vi "PH_Beckhoff_StepMot.ProcPeriodic.vi"(0 "i ref in":refnum<vi>, 3 "ms timeout (10000)":i32=10000, 5 "error in (no error)":errorcluster) -> (14 "i ref out":refnum<vi>, 17 "timed out":bool, 19 "error out":errorcluster)   [LabVIEW 2014, in "PH_Beckhoff_StepMot.lvlib"]
doc: "This method serves to periodically do things like reading values from the HW. Methods that should be executed periodically should be called from THIS methode. Add code here."
uses:
  PH_Beckhoff_StepMot.lvlib
  PH_Beckhoff/PH_Beckhoff.lvlib
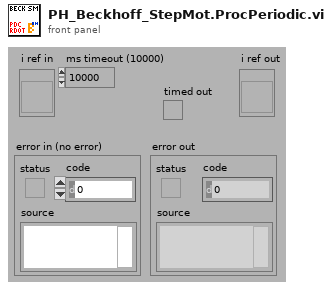
[diagram p1: front panel]
types:
  T1 = typedef "PH_Beckhoff.lvlib/PH_Beckhoff.i attribute.ctl" = cluster{"GUI Refs":T2, "operation?":bool, "Default Prdc Interval":i32, "Connection":T3, "AMS Net ID":T4, "Klemmencluster: # of":T5, "Values":T6, "IP":string, "Description":string, "configured?":bool, "Change Manager":cluster{"Detemination wanted?":bool, "Values changed at":cluster{"Sonderklemmen Inputs":i32[], "Analog Inputs":i32[], "Analog Outputs":i32[], "Digital Inputs":i32[], "Digital Outputs":i32[]}}, "Difference to handle an analog input as change":u32}
  T2 = typedef "PH_Beckhoff.lvlib/PH_Beckhoff.GUI Refs.ctl" = cluster{"ADS Error":refnum<vi>, "Values":refnum<vi>, "configured?":refnum<vi>, "Connection":refnum<vi>, "IP":refnum<vi>, "Prdc Int [ms]":refnum<vi>}
  T3 = typedef "PH_Beckhoff.lvlib/PH_Beckhoff.Connectivity.ctl" = cluster{"DLL?":bool, "Port?":bool, "Client?":bool, "Ping?":bool, "unsuccessful Pings":u32}
  T4 = typedef "Beckhoff - Driver np.lvlib/Beckhoff Access.ctl" = cluster{"DLL path":path, "AMS Net ID":cluster{"1st # of IP":u8, "2nd # of IP":u8, "3rd # of IP":u8, "4th # of IP":u8, "In Port":u8, "Out Port":u8}}
  T5 = typedef "Beckhoff - Driver np.lvlib/Klemmendeclarer.ctl" = cluster{"Offset due to Sonderklemms":u32, "analog Inputs":u32, "analog Outputs":u32, "digital Input Bits":u32, "digital Output Bits":u32}
  T6 = typedef "PH_Beckhoff.lvlib/PH_Beckhoff.Values.ctl" = cluster{"Sonderklemmen Inputs":T7, "Analog Inputs":T8, "Analog Outputs":T10, "Digital Inputs":T11, "Digital Outputs":T12}
  T7 = typedef "PH_Beckhoff.lvlib/PH_Beckhoff.Sonderklemmen Inputs.ctl" = cluster{"Total Length":u32, "Name":string, "Value":u64, "Quality":bool, "Service ID":i32, "Offset":u32, "Length":u32}[]
  T8 = typedef "PH_Beckhoff.lvlib/PH_Beckhoff.Analog Inputs.ctl" = cluster{"Name":string, "Value":u32, "Quality":bool, "Service ID":i32, "Sca Type":T9}[]
  T9 = typedef "PH_Beckhoff.lvlib/PH_Beckhoff.Scaling Type.ctl" = enum16{"none", "0 ... 15 Bit -> 0 ... 5", "0 ... 15 Bit -> 0 ... 10", "0 ... 15 Bit -> 0 ... 25", "0 ... 15 Bit -> 4 ... 20", "0 ... 15 Bit -> 0 ... 1", "0 ... 15 Bit -> 0 ... 20000", "0 ... 15 Bit -> 0 ... 24000"}
  T10 = typedef "PH_Beckhoff.lvlib/PH_Beckhoff.Analog Outputs.ctl" = cluster{"Name":string, "Value":u32, "Quality":bool, "Wanted Value":u32, "Service ID":i32, "Sca Type":T9}[]
  T11 = typedef "PH_Beckhoff.lvlib/PH_Beckhoff.Digital Inputs.ctl" = cluster{"Name":string, "Value":bool, "Quality":bool, "Service ID":i32, "inverted?":bool}[]
  T12 = typedef "PH_Beckhoff.lvlib/PH_Beckhoff.Digital Outputs.ctl" = cluster{"Name":string, "Value":bool, "Quality":bool, "Wanted Value":bool, "Service ID":i32, "inverted?":bool}[]
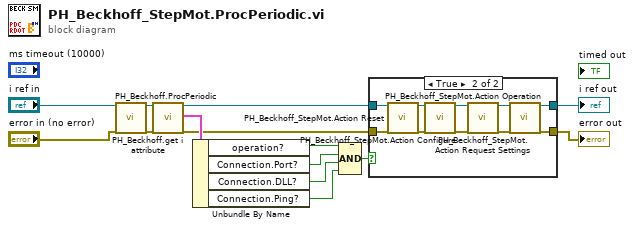
[diagram p0: block diagram]
diagram:
  n1 = call "PH_Beckhoff.ProcPeriodic.vi"("i ref in"="i ref in", "error in (no error)"="error in (no error)") -> ("i ref out"=w2:refnum<vi>, "error out"=w1:errorcluster)  [unwired: 15 in, 1 out]
  n2 = call "PH_Beckhoff.get i attribute.vi"("i ref in"=w2, "error in (no error)"=w1) -> ("i ref out"=w10:refnum<vi>, "i attribute"=w12:T1, "error out"=w9:errorcluster)  [unwired: 15 in]
  n3 = Unbundle By Name(w12) -> ("operation?"=w6:bool, "Connection.Port?"=w8:bool, "Connection.DLL?"=w7:bool, "Connection.Ping?"=w5:bool)
  n4 = Compound Arithmetic op=AND(w6, w8, w7, w5) -> (w11:bool)
  n5 = case "Constructor finished, DLL and Client found, port opened and hardware pinged?" shown="True" w11 {
    tunnel: w9 -> [w15 w26]
    tunnel: w10 -> [w16 w24]
    tunnel: [w15 w21] -> w3
    tunnel: [w16 w22] -> w4
    frame False {
    }
    frame True {
      n6 = call "PH_Beckhoff_StepMot.Action Reset.vi"("VI in"=w24, "error in (no error)"=w26) -> ("VI out"=w23:refnum<vi>, "error out"=w25:errorcluster)  [unwired: 16 in]
      n7 = call "PH_Beckhoff_StepMot.Action Configure.vi"("VI in"=w23, "error in"=w25) -> ("VI out"=w20:refnum<vi>, "error out"=w18:errorcluster)  [unwired: 16 in]
      n8 = call "PH_Beckhoff_StepMot.Action Request Settings.vi"("VI in"=w20, "error in"=w18) -> ("VI out"=w19:refnum<vi>, "error out"=w17:errorcluster)  [unwired: 16 in]
      n9 = call "PH_Beckhoff_StepMot.Action Operation.vi"("VI in"=w19, "error in"=w17) -> ("VI out"=w22:refnum<vi>, "error out"=w21:errorcluster)  [unwired: 16 in]
    }
  }
  "error out" <- w3
  "i ref out" <- w4
